vi "subImage_ApplyCursorLimit.vi"(7 "Symmetrical ROI":bool, 9 "IntGraph Refnum":refnum<vi>, 11 "Current ROI":T1={"Bin"=1, "ROI"={"x offset"=0, "y offset"=0, "x width"=2048, "y width"=2048}} {"ROI"."x offset" min=1 max=512 step=1; "ROI"."y offset" min=1 max=512 step=1; "ROI"."x width" min=1 max=512 step=1; "ROI"."y width" min=1 max=512 step=1; "Bin" items=["1x1"=1, "2x2"=2, "4x4"=4]}) -> (3 "ROI cursor":T1={"Bin"=1, "ROI"={"x offset"=0, "y offset"=0, "x width"=2048, "y width"=2048}} {"ROI"."x offset" min=1 max=512 step=1; "ROI"."y offset" min=1 max=512 step=1; "ROI"."x width" min=1 max=512 step=1; "ROI"."y width" min=1 max=512 step=1; "Bin" items=["1x1"=1, "2x2"=2, "4x4"=4]})   [LabVIEW 2015]
panel:
  # "Apply cursor limit and get ROI cursor"
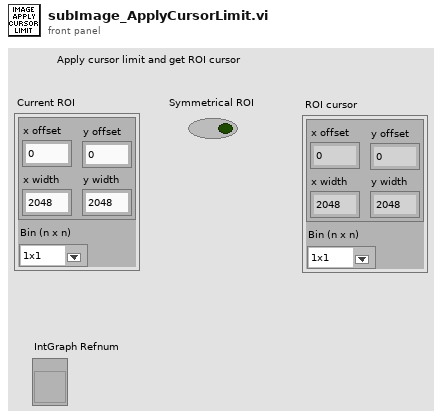
[diagram p1: front panel]
types:
  T1 = cluster{"Bin":u16, "ROI":cluster{"x offset":i32, "y offset":i32, "x width":i32, "y width":i32}}
  T2 = cluster{"x offset":i32, "y offset":i32, "x width":i32, "y width":i32}
  T3 = cluster{"x offset":dbl, "y offset":dbl, "x width":dbl, "y width":dbl}
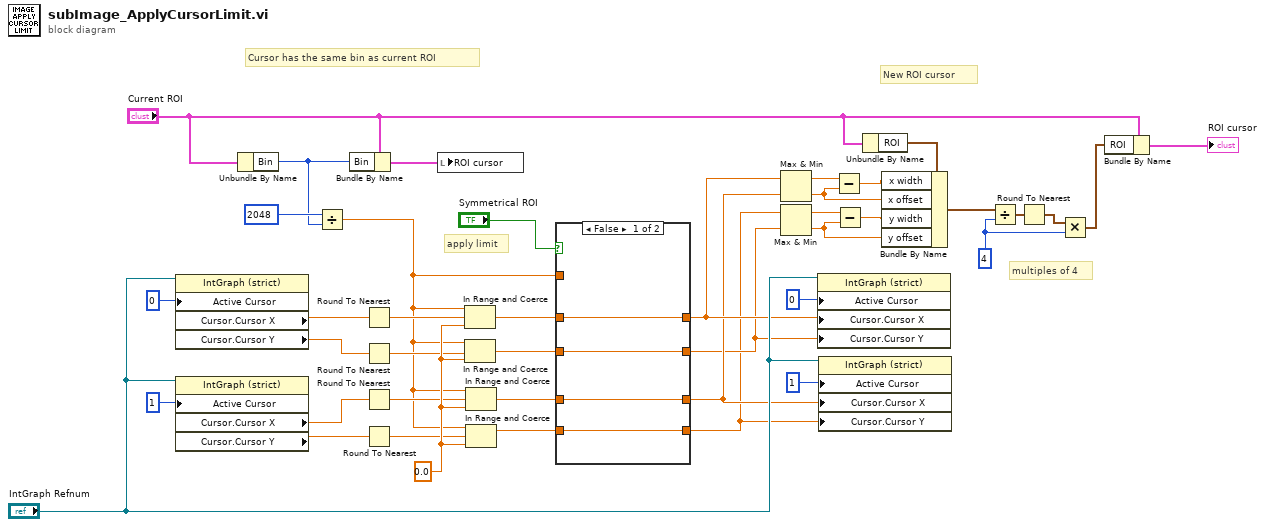
[diagram p0: block diagram]
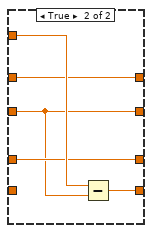
[diagram p2: hidden frame]
diagram:
  w16 = u32 4 ("Active Cursor")
  w41 = 0.0
  # "New ROI cursor"
  # "Cursor has the same bin as current ROI"
  # "multiples of 4"
  # "apply limit"
  n1 = property on="Property Node" class="IntGraph (strict)"(reference="IntGraph Refnum", "Active Cursor"=u32 0) -> ("Cursor.Cursor X"=w29:dbl, "Cursor.Cursor Y"=w28:dbl)  [unwired: 1 in, 2 out]
  n2 = property on="Property Node" class="IntGraph (strict)"(reference="IntGraph Refnum", "Active Cursor"=u32 1) -> ("Cursor.Cursor X"=w27:dbl, "Cursor.Cursor Y"=w26:dbl)  [unwired: 1 in, 2 out]
  n3 = Unbundle By Name("Current ROI") -> ("Bin"=w6:u16)
  n4 = Divide(x=u16 2048, y=w6) -> (x/y=w7:dbl)
  n5 = Bundle By Name(cluster="Current ROI", "Bin"=w6) -> (w5:T1)
  n6 = Round To Nearest(number=w29) -> (nearest integer value=w40:dbl)
  n7 = Round To Nearest(number=w28) -> (nearest integer value=w39:dbl)
  n8 = Round To Nearest(number=w27) -> (nearest integer value=w38:dbl)
  n9 = Round To Nearest(number=w26) -> (nearest integer value=w37:dbl)
  n10 = local write "ROI cursor"(w5) -> ()
  n11 = In Range and Coerce(upper limit=w7, x=w40, lower limit=w41) -> (coerced(x)=w36:dbl)  [unwired: 1 out]
  n12 = In Range and Coerce(upper limit=w7, x=w39, lower limit=w41) -> (coerced(x)=w35:dbl)  [unwired: 1 out]
  n13 = In Range and Coerce(upper limit=w7, x=w38, lower limit=w41) -> (coerced(x)=w34:dbl)  [unwired: 1 out]
  n14 = In Range and Coerce(upper limit=w7, x=w37, lower limit=w41) -> (coerced(x)=w33:dbl)  [unwired: 1 out]
  n15 = case shown="False" "Symmetrical ROI" {
    tunnel: [w45 w49] -> w12
    tunnel: w36 -> [w45 w49]
    tunnel: [w44 w46] -> w10
    tunnel: w35 -> [w44 w46]
    tunnel: [w43 w47] -> w11
    tunnel: w34 -> [w43 w47]
    tunnel: [w42 w48] -> w9
    tunnel: w33 -> [w42 _]
    tunnel: w7 -> [_ w50]
    frame False {
    }
    frame True {
      n16 = Subtract(x=w50, y=w46) -> (x-y=w48:dbl)
    }
  }
  n17 = Max & Min(x=w12, y=w11) -> (max(x,y)=w22:dbl, min(x,y)=w19:dbl)
  n18 = Max & Min(x=w9, y=w10) -> (max(x,y)=w21:dbl, min(x,y)=w17:dbl)
  n19 = property on="Property Node" class="IntGraph (strict)"(reference="IntGraph Refnum", "Active Cursor"=u32 0, "Cursor.Cursor X"=w12, "Cursor.Cursor Y"=w10) -> ()  [unwired: 1 in, 2 out]
  n20 = property on="Property Node" class="IntGraph (strict)"(reference="IntGraph Refnum", "Active Cursor"=u32 1, "Cursor.Cursor X"=w11, "Cursor.Cursor Y"=w9) -> ()  [unwired: 1 in, 2 out]
  n21 = Subtract(x=w22, y=w19) -> (x-y=w20:dbl)
  n22 = Subtract(x=w21, y=w17) -> (x-y=w18:dbl)
  n23 = Unbundle By Name("Current ROI") -> ("ROI"=w4:T2)
  n24 = Bundle By Name(cluster=w4, "x width"=w20, "x offset"=w19, "y width"=w18, "y offset"=w17) -> (w13:T2)
  n25 = Divide(x=w13, y=w16) -> (x/y=w14:T3)
  n26 = Round To Nearest(number=w14) -> (nearest integer value=w15:T3)
  n27 = Multiply(x=w15, y=w16) -> (x*y=w1:T3)
  n28 = Bundle By Name(cluster="Current ROI", "ROI"=w1) -> (→"ROI cursor":T1)
